vi "ReadObjectLayout.vi"(7 "properties to ignore":variant, 8 "error in (no error)":errorcluster, 10 "GObj Refnum":refnum<vi>, 11 "XControl Layout in":refnum<class "XControl Layout.lvclass">) -> (0 "error out":errorcluster, 3 "XControl Layout out":refnum<class "XControl Layout.lvclass">)   [LabVIEW 2010, in "NI_SE_Front Panel Layout.lvlib" / "XControl Layout.lvclass"]
doc: "Read layout information from the GObj Refnum."
uses:
  XControl Layout.lvclass
  Control Layout/Control Layout.lvclass
  XControl Layout.lvclass/XControl Layout.ctl
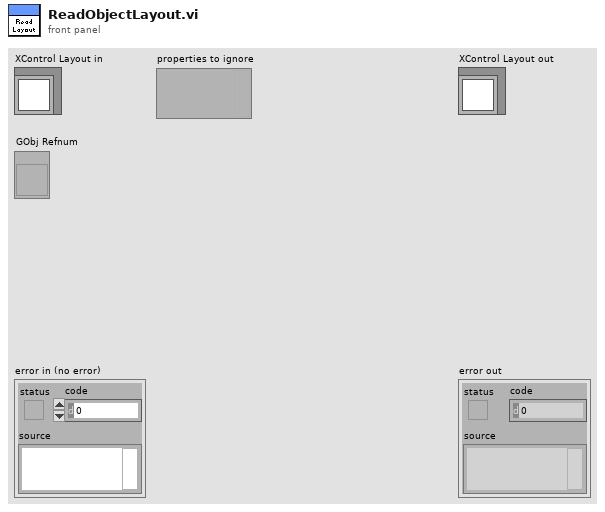
[diagram p1: front panel]
types:
  T1 = typedef "LVBoundsTypeDef.ctl" = cluster{"Width":u32, "Height":u32}
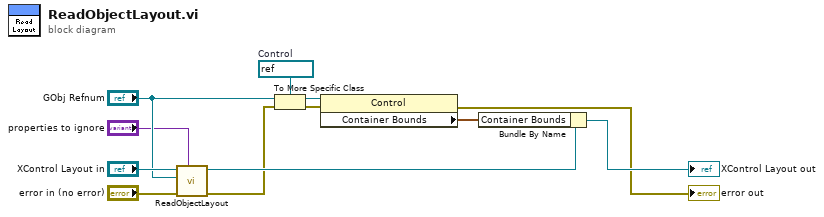
[diagram p0: block diagram]
diagram:
  w4 = refnum<vi> refnum  # Control
  n1 = call-parent "ReadObjectLayout.vi"("properties to ignore"="properties to ignore", "error in (no error)"="error in (no error)", "GObj Refnum"="GObj Refnum", "Control Layout in"="XControl Layout in") -> ("error out"=w9:errorcluster, "Control Layout out"=w10:refnum<class "XControl Layout.lvclass">)  [unwired: 6 in]
  n2 = To More Specific Class(target class=w4, reference="GObj Refnum", error in=w9) -> (specific class reference=w3:refnum<vi>, error out=w2:errorcluster)
  n3 = property class="Control"(reference=w3, error in=w2) -> (error out=→"error out":errorcluster, "Container Bounds"=w1:T1)  [unwired: 1 out]
  n4 = Bundle By Name(cluster=w10, "Container Bounds"=w1) -> (→"XControl Layout out":refnum<class "XControl Layout.lvclass">)
